vi "Get Valid Properties.vi"(8 "error in (no error)":errorcluster, 11 "ToneCloud in":refnum<class "Tone Cloud.lvclass">) -> (0 "error out":errorcluster, 2 "Properties":string[](array[string]), 3 "ToneCloud out":refnum<class "Tone Cloud.lvclass">)   [LabVIEW 2020, in "Tone Cloud.lvclass"]
uses:
  Tone Cloud.lvclass
  Tone Cloud.lvclass/Tone Cloud.ctl
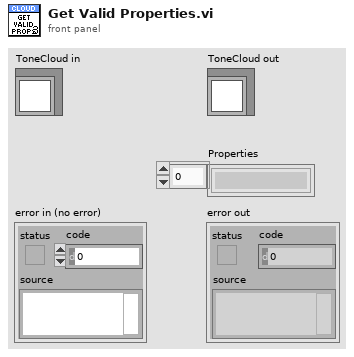
[diagram p1: front panel]
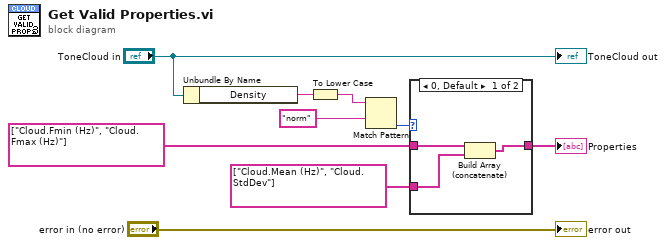
[diagram p0: block diagram]
diagram:
  n1 = Unbundle By Name("ToneCloud in") -> ("Density"=w7:string)
  n2 = To Lower Case(string=w7) -> (all lower case string=w5:string)
  n3 = Match Pattern(string=w5, regular expression="norm") -> (offset past match=w3:i32)  [unwired: 1 in, 3 out]
  n4 = case shown="0, Default" w3 {
    tunnel: string[] ["Cloud.Fmin (Hz)", "Cloud.Fmax (Hz)"] ("Properties") -> [w12 w13]
    tunnel: [w11 w13] -> w2
    tunnel: string[] ["Cloud.Mean (Hz)", "Cloud.StdDev"] ("Properties") -> [w10 _]
    frame 0, Default {
      n5 = Build Array (concatenate)(w12, w10) -> (w11:string[])
    }
    frame -1 {
    }
  }
  "Properties" <- w2
  "error out" <- "error in (no error)"
  "ToneCloud out" <- "ToneCloud in"
